vi "LWXPS_PositionerCorrectorPIDFFAccelerationGet.vi"(0 "XPS Reference IN":refnum<k24>, 2 "Positioner Name":string, 7 "LabVIEW error IN":errorcluster) -> (11 "LabVIEW error OUT":errorcluster, 12 "XPS Reference OUT":refnum<k24>, 13 "XPS Error String":string, 14 "Returned error code":i32, 15 "Feed Forward jerk":dbl, 16 "Closed Loop Status":bool, 17 "Feed forward acceleration":dbl, 18 "Proportional gain":dbl, 19 "Form coefficient":dbl, 20 "Integral gain":dbl, 21 "Derivative gain":dbl, 22 "Integral saturation value":dbl, 23 "Integration time":dbl, 24 "Derivative filter cut off frequency":dbl, 25 "Proportional gain multiplier":dbl, 26 "Integral gain multiplier":dbl, 27 "Derivative gain multiplier":dbl)   [LabVIEW 2014]
uses:
  D:/XPSQ8_LabView_Library/Development/Source/Dll/Newport.XPS.CommandInterface.dll
  Dll/Newport.XPS.CommandInterface.dll
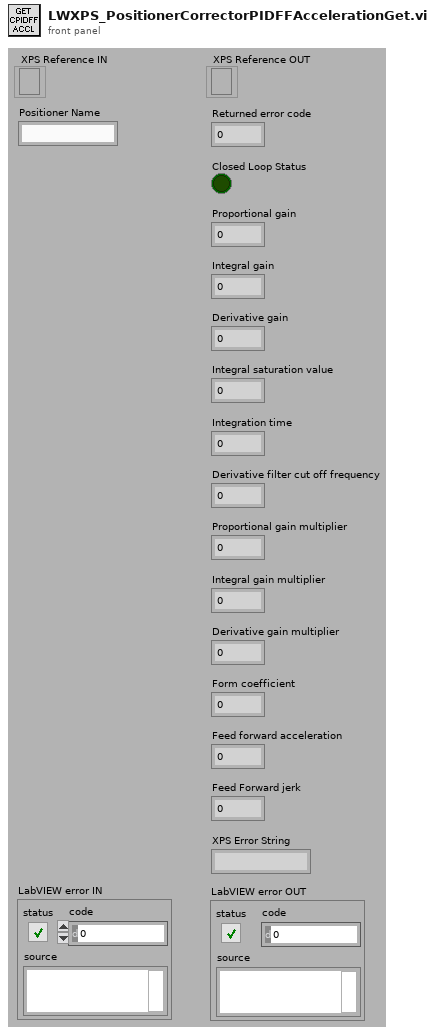
[diagram p1: front panel]
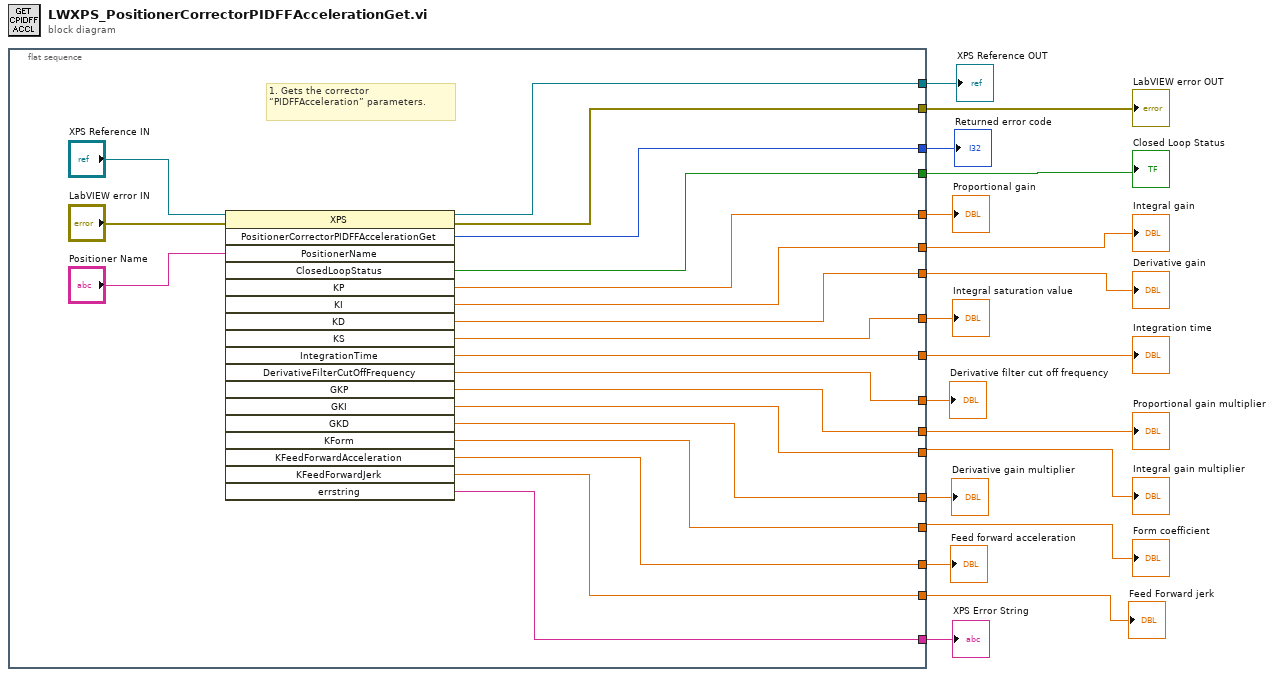
[diagram p0: block diagram]
diagram:
  n1 = flat-sequence {
    tunnel: [w35] -> w7
    tunnel: [w28] -> w17
    tunnel: [w36] -> w16
    tunnel: [w32] -> w15
    tunnel: [w31] -> w14
    tunnel: [w29] -> w13
    tunnel: [w30] -> w12
    tunnel: [w23] -> w11
    tunnel: [w27] -> w8
    tunnel: [w26] -> w10
    tunnel: [w25] -> w9
    tunnel: [w24] -> w2
    tunnel: [w22] -> w6
    tunnel: [w21] -> w5
    tunnel: [w20] -> w4
    tunnel: [w19] -> w3
    tunnel: [w18] -> w1
    frame #0 {
      # "1. Gets the corrector “PIDFFAcceleration” parameters."
      n2 = invoke class="XPS" method="PositionerCorrectorPIDFFAccelerationGet"(reference="XPS Reference IN", error in="LabVIEW error IN", "PositionerName"="Positioner Name") -> (reference out=w35:refnum<k24>, error out=w28:errorcluster, "PositionerCorrectorPIDFFAccelerationGet"=w36:i32, "ClosedLoopStatus"=w27:bool, "KP"=w32:dbl, "KI"=w31:dbl, "KD"=w29:dbl, "KS"=w30:dbl, "IntegrationTime"=w23:dbl, "DerivativeFilterCutOffFrequency"=w26:dbl, "GKP"=w25:dbl, "GKI"=w24:dbl, "GKD"=w22:dbl, "KForm"=w21:dbl, "KFeedForwardAcceleration"=w20:dbl, "KFeedForwardJerk"=w19:dbl, "errstring"=w18:string)  [unwired: 15 in, 1 out]
    }
  }
  "XPS Error String" <- w1
  "XPS Reference OUT" <- w7
  "LabVIEW error OUT" <- w17
  "Returned error code" <- w16
  "Proportional gain" <- w15
  "Integral gain" <- w14
  "Derivative gain" <- w13
  "Integral saturation value" <- w12
  "Integration time" <- w11
  "Derivative filter cut off frequency" <- w10
  "Proportional gain multiplier" <- w9
  "Closed Loop Status" <- w8
  "Derivative gain multiplier" <- w6
  "Form coefficient" <- w5
  "Feed forward acceleration" <- w4
  "Feed Forward jerk" <- w3
  "Integral gain multiplier" <- w2
